vi "MsgMyMessage.vi"() -> (1 "MessageName":string)   [LabVIEW 2017, in "Loop8.lvlib"]
uses:
  <vilib>/addons/InsightCM/Devices/Shared/Common/DataFlow/test/SpeedBenchmark/Loop8/Loop8.lvlib
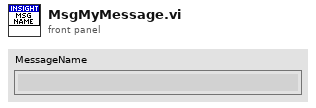
[diagram p1: front panel]
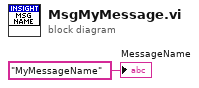
[diagram p0: block diagram]
diagram:
  "MessageName" <- "MyMessageName" ("ProcessName")
